vi "ReadSwerveSensors.vi"(5 "BR Desired Position":dbl, 7 "BR Throttle":dbl) -> ()   [LabVIEW 2020]
panel:
  in  "Recording":bool
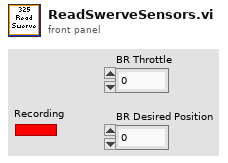
[diagram p1: front panel]
types:
  T1 = enum16{"open", "replace", "create", "open or create", "replace or create", "replace or create with confirmation"}
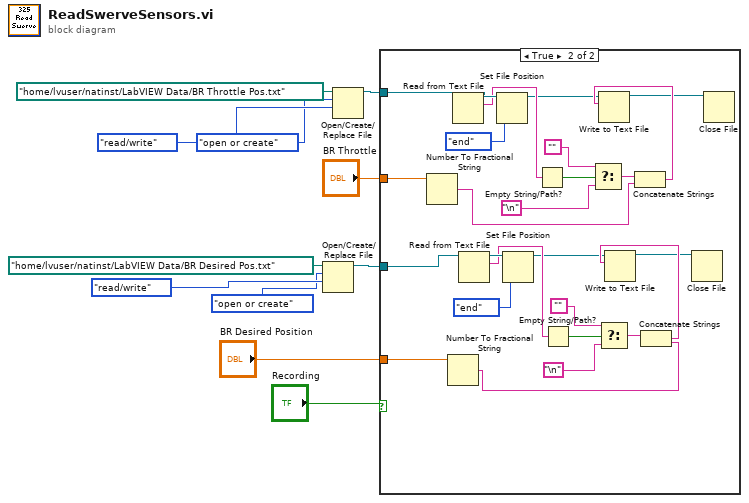
[diagram p0: block diagram]
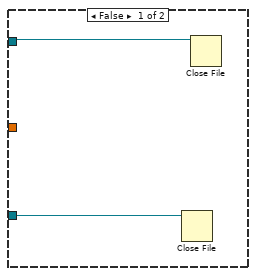
[diagram p2: hidden frame]
diagram:
  n1 = Open/Create/Replace File(file path (use dialog)=path "/home/lvuser/natinst/LabVIEW Data/BR Desired Pos.txt", operation (0:open)=T1."open or create", access (0:read/write)=enum16{"read/write", "read-only", "write-only"}."read/write") -> (refnum out=w8:refnum<file>)  [unwired: 3 in, 2 out]
  n2 = Open/Create/Replace File(file path (use dialog)=path "/home/lvuser/natinst/LabVIEW Data/BR Throttle Pos.txt", operation (0:open)=T1."open or create", access (0:read/write)=enum16{"read/write", "read-only", "write-only"}."read/write") -> (refnum out=w7:refnum<file>)  [unwired: 3 in, 2 out]
  n3 = case shown="True" "Recording" {
    tunnel: w8 -> [w12 w29]
    tunnel: "BR Desired Position" -> [_ w27]
    tunnel: w7 -> [w13 w16]
    tunnel: "BR Throttle" -> [_ w14]
    frame False {
      n4 = Close File(refnum=w12) -> ()  [unwired: 1 in, 2 out]
      n5 = Close File(refnum=w13) -> ()  [unwired: 1 in, 2 out]
    }
    frame True {
      n6 = Number To Fractional String(number=w14) -> (F-format string=w15:string)  [unwired: 3 in]
      n7 = Number To Fractional String(number=w27) -> (F-format string=w33:string)  [unwired: 3 in]
      n8 = Read from Text File(file (use dialog)=w16) -> (refnum out=w26:refnum<file>, text=w19:string)  [unwired: 3 in, 2 out]
      n9 = Read from Text File(file (use dialog)=w29) -> (refnum out=w39:refnum<file>, text=w31:string)  [unwired: 3 in, 2 out]
      n10 = Set File Position(refnum=w26, from (0:start)=enum16{"start", "end", "current"}."end") -> (refnum out=w18:refnum<file>)  [unwired: 2 in, 1 out]
      n11 = Set File Position(refnum=w39, from (0:start)=enum16{"start", "end", "current"}."end") -> (refnum out=w30:refnum<file>)  [unwired: 2 in, 1 out]
      n12 = Empty String/Path?(string/path=w19) -> (empty?=w24:bool)
      n13 = Empty String/Path?(string/path=w31) -> (empty?=w37:bool)
      n14 = Select(t="", s=w24, f="\n") -> (s? t:f=w21:string)
      n15 = Select(t="", s=w37, f="\n") -> (s? t:f=w34:string)
      n16 = Concatenate Strings(w21, w15) -> (w20:string)
      n17 = Write to Text File(file (use dialog)=w18, text=w20) -> (refnum out=w17:refnum<file>)  [unwired: 2 in, 2 out]
      n18 = Concatenate Strings(w34, w33) -> (w32:string)
      n19 = Write to Text File(file (use dialog)=w30, text=w32) -> (refnum out=w28:refnum<file>)  [unwired: 2 in, 2 out]
      n20 = Close File(refnum=w28) -> ()  [unwired: 1 in, 2 out]
      n21 = Close File(refnum=w17) -> ()  [unwired: 1 in, 2 out]
    }
  }
